vi "Analyzer.vi"() -> ()   [LabVIEW 2015]
panel:
  out "Waveform Graph":i32[][](graph)
  out "t":i32[](array[numeric])
  out "z":i32[](array[numeric])
  out "y":i32[](array[numeric])
  out "x":i32[](array[numeric])
  in  "filePath":path
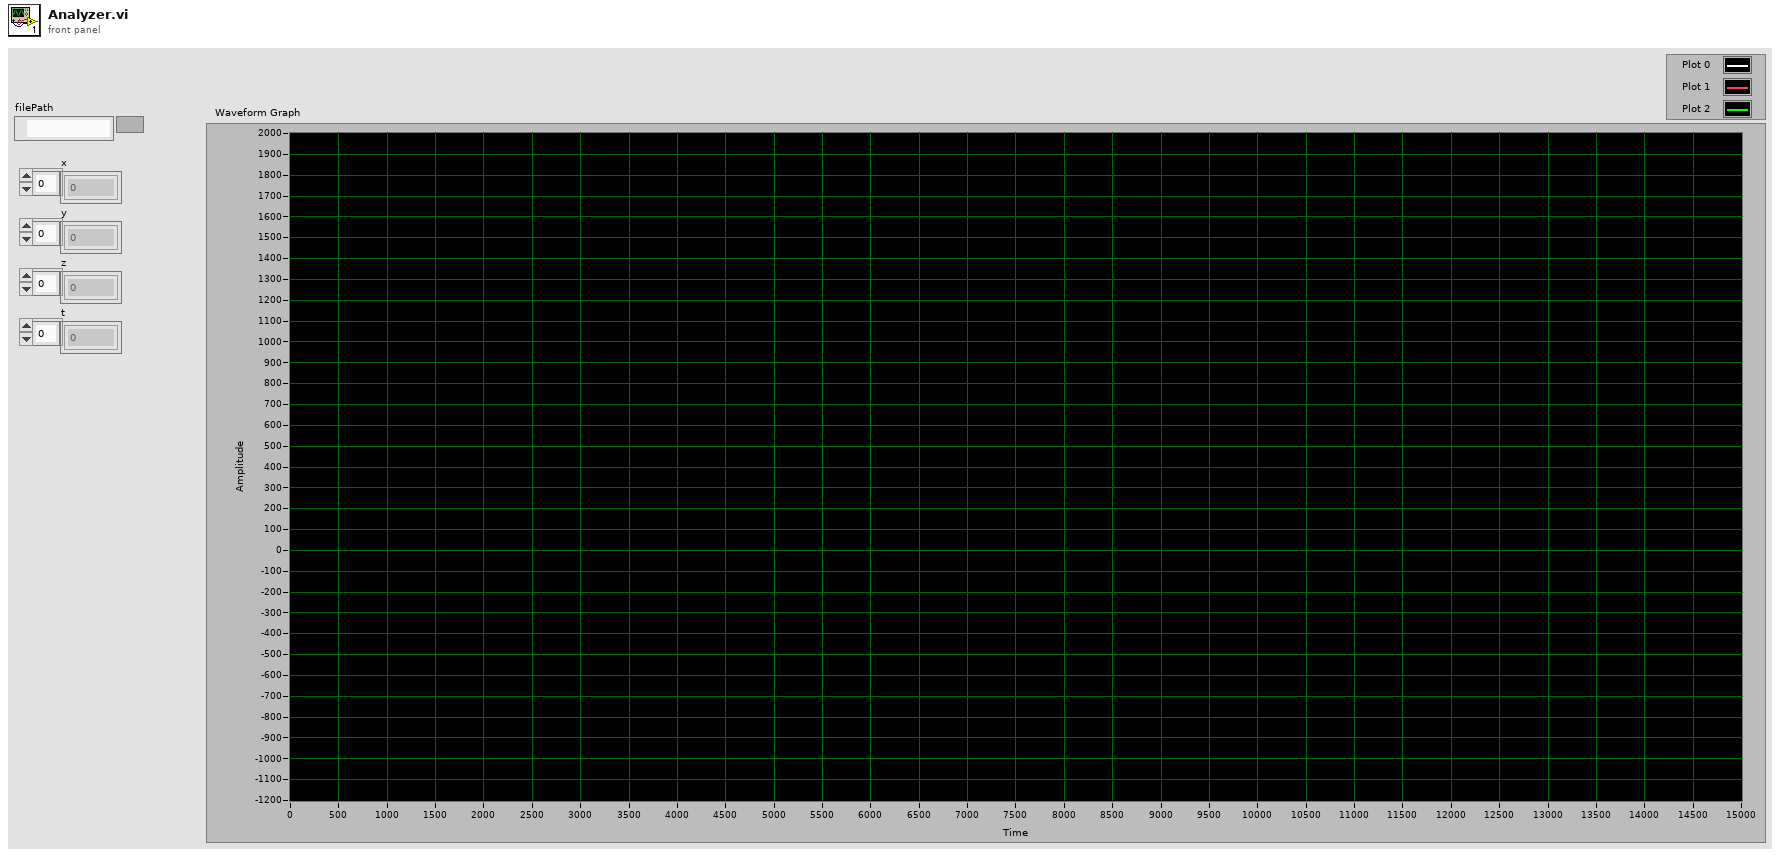
[diagram p1: front panel]
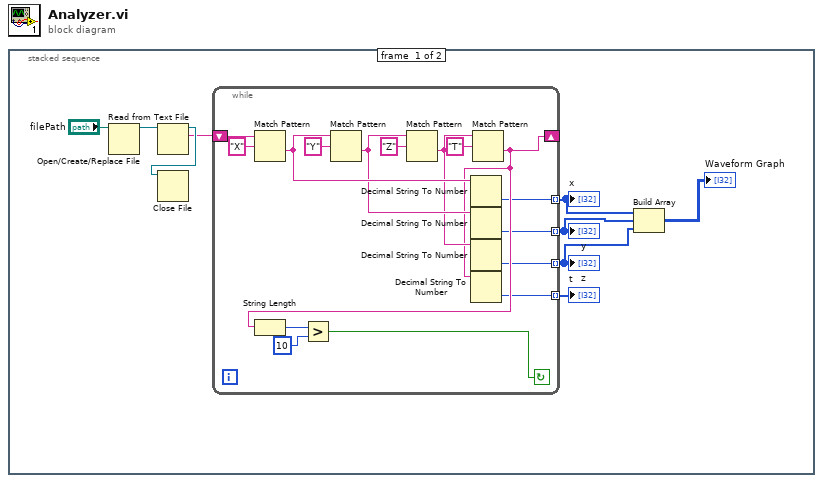
[diagram p0: block diagram]
diagram:
  n1 = stacked-sequence {
    frame #0 {
      n2 = Open/Create/Replace File(file path (use dialog)="filePath") -> (refnum out=w8:refnum<file>)  [unwired: 5 in, 2 out]
      n3 = Read from Text File(file (use dialog)=w8) -> (refnum out=w7:refnum<file>, text=w6:string)  [unwired: 3 in, 2 out]
      n4 = Close File(refnum=w7) -> ()  [unwired: 1 in, 2 out]
      n5 = while {
        shift-right: [w17] -> _
        shift-left: w6 -> [w20]
        tunnel: [w16] -> w4 mode=indexing
        tunnel: [w15] -> w3 mode=indexing
        tunnel: [w14] -> w2 mode=indexing
        tunnel: [w13] -> w5 mode=indexing
        stop <- w10 continue-if-true
        n6 = Match Pattern(string=w20, regular expression="X") -> (after substring=w21:string)  [unwired: 1 in, 3 out]
        n7 = Match Pattern(string=w21, regular expression="Y") -> (after substring=w19:string)  [unwired: 1 in, 3 out]
        n8 = Match Pattern(string=w19, regular expression="Z") -> (after substring=w18:string)  [unwired: 1 in, 3 out]
        n9 = Decimal String To Number(string=w21) -> (number=w16:i32)  [unwired: 2 in, 1 out]
        n10 = Decimal String To Number(string=w19) -> (number=w15:i32)  [unwired: 2 in, 1 out]
        n11 = Decimal String To Number(string=w18) -> (number=w14:i32)  [unwired: 2 in, 1 out]
        n12 = Match Pattern(string=w18, regular expression="T") -> (after substring=w17:string)  [unwired: 1 in, 3 out]
        n13 = String Length(string=w17) -> (length=w12:i32)
        n14 = Greater?(x=w12, y=10) -> (0:w10:bool)
        n15 = Decimal String To Number(string=w17) -> (number=w13:i32)  [unwired: 2 in, 1 out]
      }
      "x" <- w4
      "y" <- w3
      "z" <- w2
      "t" <- w5
      n16 = Build Array(w4, w3, w2) -> (→"Waveform Graph":i32[][])
    }
    frame #1 {
    }
  }
